vi "set_H2N2_display.vi"(0 "Manifold N2 Flow":dbl, 1 "Manifold H2 Flow":dbl, 2 "Display H2 or N2":bool, 3 "H2 Active":bool, 4 "N2 Active":bool, 5 "Remote":bool) -> ()   [LabVIEW 2011]
uses:
  low_level_proc/globals.vi
  editor_lib/Flow_Globals.vi
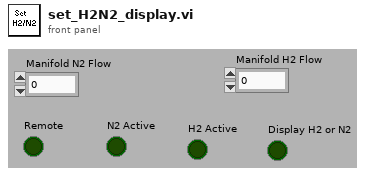
[diagram p1: front panel]
types:
  T1 = typedef "relaySpec.ctl" = cluster{"Card Index":u16, "Relay Index":u16}
  T2 = typedef "DA_Spec.ctl" = cluster{"Card Index":u16, "Channel Index":u16}
  T3 = typedef "AD_Spec.ctl" = u16
  T4 = cluster{"Relay Functions":cluster{"Remote":T1, "H2 active":T1, "N2 active":T1, "Output":T1}, "D/A Functions":cluster{"H2 flow":T2, "N2 flow":T2}, "Flow Ranges":cluster{"H2 flow (HMFC1)":u16, "N2 flow (NMFC1)":u16}, "A/D Functions":cluster{"H2/N2 flow":T3}}
  T5 = cluster{"Remote":T1, "H2 active":T1, "N2 active":T1, "Output":T1}
  T6 = cluster{"H2 flow (HMFC1)":u16, "N2 flow (NMFC1)":u16}
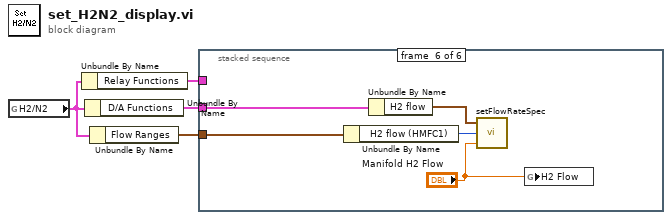
[diagram p0: block diagram]
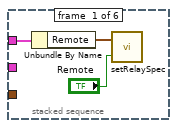
[diagram p2: hidden frame]
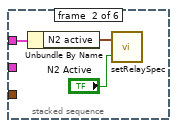
[diagram p3: hidden frame]
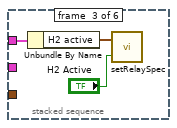
[diagram p4: hidden frame]
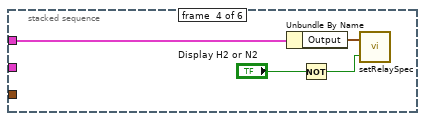
[diagram p5: hidden frame]
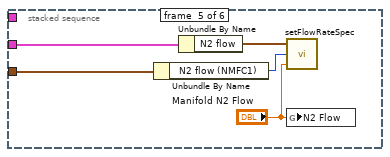
[diagram p6: hidden frame]
diagram:
  n1 = global read "globals.vi" "H2/N2"() -> (w2:T4)
  n2 = Unbundle By Name(w2) -> ("Relay Functions"=w4:T5)
  n3 = Unbundle By Name(w2) -> ("D/A Functions"=w3:cluster{"H2 flow":T2, "N2 flow":T2})
  n4 = Unbundle By Name(w2) -> ("Flow Ranges"=w1:T6)
  n5 = stacked-sequence {
    tunnel: w4 -> [w7 w10 w12 w16 _ _]
    tunnel: w3 -> [_ _ _ _ w21 w25]
    tunnel: w1 -> [_ _ _ _ w19 w27]
    frame #0 {
      n6 = Unbundle By Name(w7) -> ("Remote"=w6:T1)
      n7 = call "setRelaySpec.vi"("Relay Status"="Remote", "RelaySpec"=w6) -> ()  [unwired: 1 in]
    }
    frame #1 {
      n8 = Unbundle By Name(w10) -> ("N2 active"=w9:T1)
      n9 = call "setRelaySpec.vi"("Relay Status"="N2 Active", "RelaySpec"=w9) -> ()  [unwired: 1 in]
    }
    frame #2 {
      n10 = Unbundle By Name(w12) -> ("H2 active"=w11:T1)
      n11 = call "setRelaySpec.vi"("Relay Status"="H2 Active", "RelaySpec"=w11) -> ()  [unwired: 1 in]
    }
    frame #3 {
      n12 = Unbundle By Name(w16) -> ("Output"=w15:T1)
      n13 = Not(x="Display H2 or N2") -> (.not. x?=w14:bool)
      n14 = call "setRelaySpec.vi"("Relay Status"=w14, "RelaySpec"=w15) -> ()  [unwired: 1 in]
    }
    frame #4 {
      n15 = Unbundle By Name(w19) -> ("N2 flow (NMFC1)"=w18:u16)
      n16 = Unbundle By Name(w21) -> ("N2 flow"=w20:T2)
      n17 = call "setFlowRateSpec.vi"("Flow Rate (sccm)"="Manifold N2 Flow", "Flow range Index"=w18, "D/A Card"=w20) -> ()  [unwired: 2 in]
      n18 = global write "Flow_Globals.vi" "N2 Flow"("Manifold N2 Flow") -> ()
    }
    frame #5 {
      n19 = Unbundle By Name(w27) -> ("H2 flow (HMFC1)"=w26:u16)
      n20 = Unbundle By Name(w25) -> ("H2 flow"=w24:T2)
      n21 = call "setFlowRateSpec.vi"("Flow Rate (sccm)"="Manifold H2 Flow", "Flow range Index"=w26, "D/A Card"=w24) -> ()  [unwired: 2 in]
      n22 = global write "Flow_Globals.vi" "H2 Flow"("Manifold H2 Flow") -> ()
    }
  }
